vi "OSA20X_GetAttributes.vi"(0 "reference in":refnum<class "OSA.lvclass">, 1 "OnlyGetDvrReference(False)":bool, 5 "error in (no error)":errorcluster) -> (14 "reference out":refnum<class "OSA.lvclass">, 15 "Data":T1={"Stop"=FALSE, "dataType"=enum."interferogram", "spectrometerIdx"=0, "buffer size interferogram"=0, "interferogram"={"new"=FALSE, "plot_x_ min"=0.0, "plot_x_max"=0.0, "plot_y_min"=0.0, "plot_y_max"=0.0, "Graph Intrfrgrm"=refnum, "timeStamp"=0, "signal (%)"=0.0, "traces"=[], "traces idx last"=0}, "spectrum"={"new"=FALSE, "plot_x_min"=0.0, "plot_x_max"=0.0, "plot_unit_x"=enum."wavenr/cm", "plot_unit_y"=enum."ADC counts", "plot_y_min"=0.0, "plot_y_max"=0.0, "Graph Spectrum"=refnum, "timeStamp"=0, "X_VAL_OPTIONS"=enum."MIN_MAX", "traces"=[], "traces idx last"=0}, "Thorlabs_OSA_64.lvclass:queue_action.ctlqueue ref"=refnum, "action"=enum."none", "plot zoom step"=0.0, "buffer semaphore"=refnum, "acq stopped"=FALSE, "dataType active"=enum."interferogram", "temperature (degr C)"=0.0, "pressure (hPa)"=0.0, "rel humidity (%)"=0.0, "settings"={"resolution"=0, "sensitivity"=0, "Average"=FALSE, "average nr"=1, "apodisation"=enum."NONE", "acq delay (ms)"=500, "airMesure"=enum."TEMPERATURE", "wmtr on"=FALSE, "intfgrm_smooth_width"=0, "intfgrm_smooth_nrOfPasses"=0, "intfgrm_smooth"=enum."NONE", "phaseCorrection"=enum."NONE", "zeroFill"=0, "spectr_smooth"=enum."NONE", "spectr_smooth_width"=0, "spectr_smooth_nrOfPasses"=0, "resolution (/cm)"=0.0, "REF wavelength, (nm)"=0.0, "gain_idx"=0, "gainAuto"=FALSE, "gain_relative"=0.0, "PD sensitivity mode"=enum."cool: better sensitivity/noise floor", "PD senseMode implemented"=FALSE, "SensorTemperature implemented"=FALSE, "SensorPressure implemented"=FALSE, "SensorHumidity implemented"=FALSE, "attenuationAuto"=FALSE, "attenuationOnOff"=FALSE, "attenuationAvailable"=FALSE, "offsetAvailable"=FALSE, "offset"=0, "offset max"=0}, "peaks position"=[], "peaks width"=[], "peaks height"=[], "peaks max nr"=0, "peaks latest nr"=0, "peaks new"=FALSE, "power"=0.0, "power new"=FALSE, "path"="", "wavelength (WNr)"=0.0, "wavelength new"=FALSE, "buffer size spectrum"=0, "status"="", "vi reference"=refnum, "funcPointer"=0, "libraryPointer"=0, "singleAcquisition"=FALSE, "coherenceLength (cm)"=0.0, "coherenceLength new"=FALSE, "spectrometer model"="", "spectrometer serial nr"="", "peaks thld left"=[], "peaks thld right"=[], "coherenceLength error (cm)"=0.0, "ADC bits"=0, "peaks position centroid"=[], "peaks height centroid"=[], "OSA series"=enum."OSA200", "channel index spectrum"=0, "spectrometer rangeLow, (/cm)"=0.0, "spectrometer rangeHigh, (/cm)"=0.0, "channel index interferogram"=0} {"peaks height centroid" format="%.2f"; "peaks position centroid" format="%.2f"; "coherenceLength error (cm)" format="%.2f"; "peaks thld right" format="%.2f"; "peaks thld left" format="%.2f"; "coherenceLength (cm)" format="%.2f"; "wavelength (WNr)" format="%.2f"; "power" format="%.2f"; "peaks height" format="%.2f"; "peaks width" format="%.2f"; "peaks position" format="%.2f"; "settings"."REF wavelength, (nm)" format="%.2f"; "settings"."resolution (/cm)" format="%.2f"; "settings"."acq delay (ms)" step=200; "settings"."average nr" min=1 max=100 step=1; "rel humidity (%)" format="%.2f"; "pressure (hPa)" format="%.2f"; "temperature (degr C)" format="%.2f"; "plot zoom step" format="%.2f"; "spectrum"."plot_y_max" format="%.2f"; "spectrum"."plot_y_min" format="%.2f"; "spectrum"."plot_x_max" format="%.2f"; "spectrum"."plot_x_min" format="%.2f"; "interferogram"."plot_y_max" format="%.2f"; "interferogram"."plot_y_min" format="%.2f"; "interferogram"."plot_x_max" format="%.2f"; "interferogram"."plot_x_ min" format="%.2f"}, 17 "DataRef":refnum<data-value>, 19 "error out":errorcluster)   [LabVIEW 2010, in "OSA.lvclass"]
uses:
  OSA.lvclass
  protected/ObjectAttributes.ctl
  typeDef/acq_dataType.ctl
  private/graph_intensity.ctl
  typeDef/spectrum_x_unit.ctl
  typeDef/y_unit.ctl
  misc_examples/action_data.ctl
  typeDef/queue_action.ctl
  typeDef/apodisation.ctl
  typeDef/airMeasure.ctl
  _misc/Thorlabs_FTS_misc.llb/interferogram_smoothing.ctl
  typeDef/phaseCorrection.ctl
  _misc/Thorlabs_FTS_misc.llb/PDTemperatureMode.ctl
  typeDef/OSA_series.ctl
  OSA.lvclass/OSA.ctl
  OSA20X_misc.lvlib
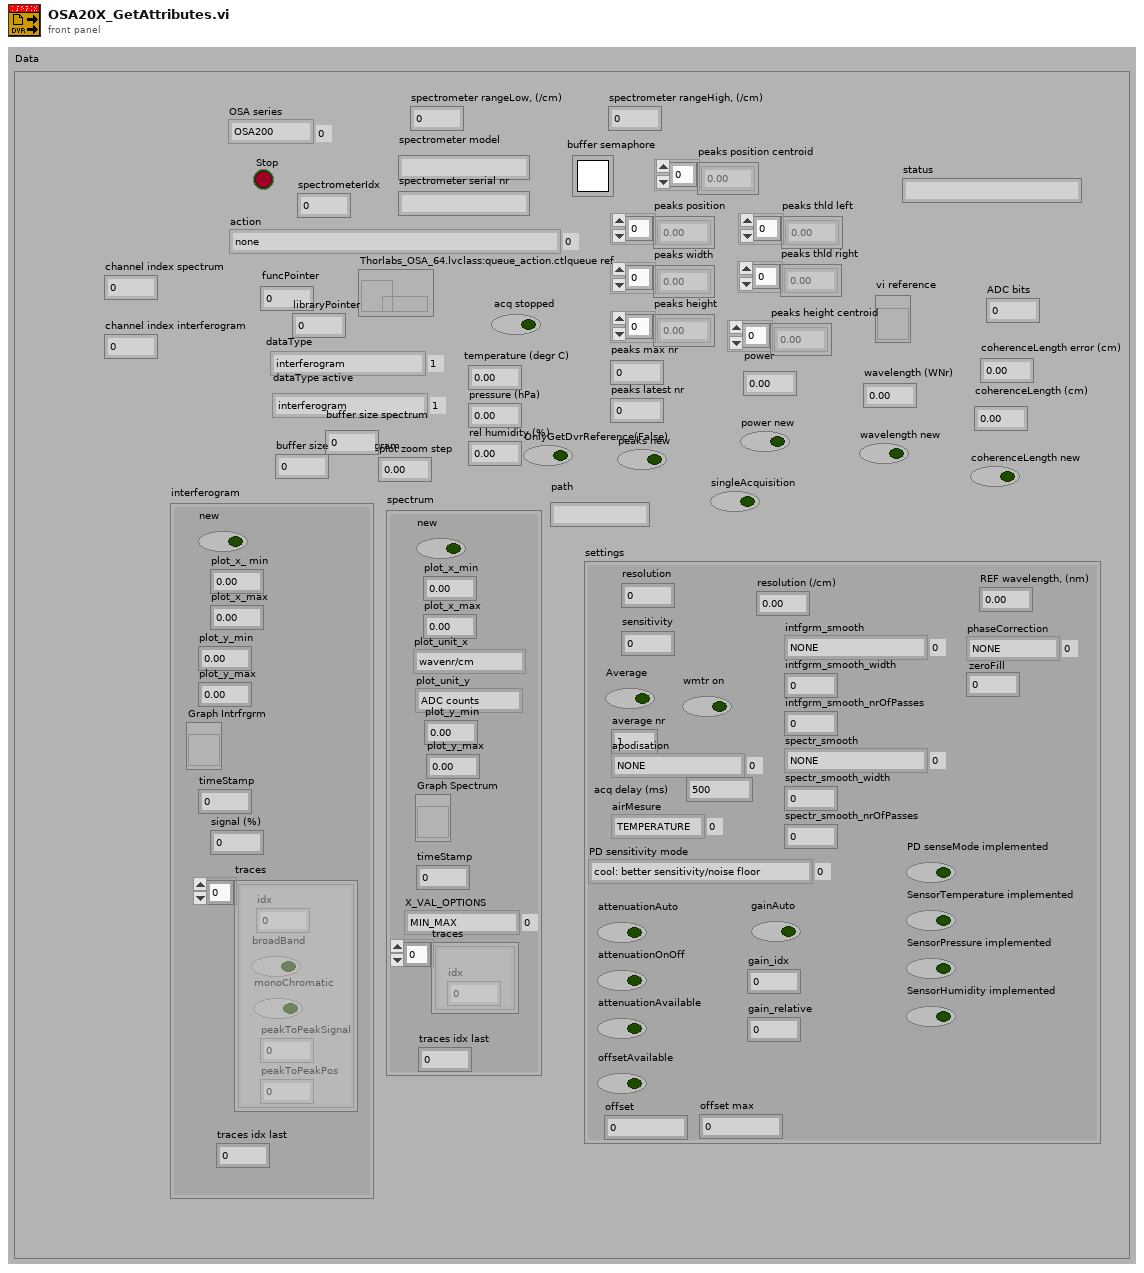
[diagram p1: front panel]
types:
  T1 = typedef "OSA.lvclass/ObjectAttributes.ctl" = cluster{"Stop":bool, "dataType":T2, "spectrometerIdx":u16, "buffer size interferogram":i32, "interferogram":cluster{"new":bool, "plot_x_ min":sgl, "plot_x_max":sgl, "plot_y_min":sgl, "plot_y_max":sgl, "Graph Intrfrgrm":T3, "timeStamp":u32, "signal (%)":dbl, "traces":cluster{"idx":u32, "broadBand":bool, "monoChromatic":bool, "peakToPeakSignal":dbl, "peakToPeakPos":dbl}[], "traces idx last":i32}, "spectrum":cluster{"new":bool, "plot_x_min":sgl, "plot_x_max":sgl, "plot_unit_x":T4, "plot_unit_y":T5, "plot_y_min":sgl, "plot_y_max":sgl, "Graph Spectrum":T3, "timeStamp":u32, "X_VAL_OPTIONS":enum16{"MIN_MAX", "ARRAY"}, "traces":cluster{"idx":u32}[], "traces idx last":i32}, "Thorlabs_OSA_64.lvclass:queue_action.ctlqueue ref":refnum<queue>, "action":T6, "plot zoom step":dbl, "buffer semaphore":T7, "acq stopped":bool, "dataType active":T2, "temperature (degr C)":sgl, "pressure (hPa)":sgl, "rel humidity (%)":sgl, "settings":cluster{"resolution":u16, "sensitivity":u16, "Average":bool, "average nr":u32, "apodisation":T8, "acq delay (ms)":u32, "airMesure":T9, "wmtr on":bool, "intfgrm_smooth_width":u16, "intfgrm_smooth_nrOfPasses":u16, "intfgrm_smooth":T10, "phaseCorrection":T11, "zeroFill":u8, "spectr_smooth":T10, "spectr_smooth_width":u16, "spectr_smooth_nrOfPasses":u16, "resolution (/cm)":sgl, "REF wavelength, (nm)":dbl, "gain_idx":u16, "gainAuto":bool, "gain_relative":dbl, "PD sensitivity mode":T12, "PD senseMode implemented":bool, "SensorTemperature implemented":bool, "SensorPressure implemented":bool, "SensorHumidity implemented":bool, "attenuationAuto":bool, "attenuationOnOff":bool, "attenuationAvailable":bool, "offsetAvailable":bool, "offset":i32, "offset max":u16}, "peaks position":sgl[], "peaks width":sgl[], "peaks height":sgl[], "peaks max nr":u32, "peaks latest nr":i32, "peaks new":bool, "power":dbl, "power new":bool, "path":string, "wavelength (WNr)":dbl, "wavelength new":bool, "buffer size spectrum":i32, "status":string, "vi reference":refnum<vi>, "funcPointer":u64, "libraryPointer":u64, "singleAcquisition":bool, "coherenceLength (cm)":dbl, "coherenceLength new":bool, "spectrometer model":string, "spectrometer serial nr":string, "peaks thld left":sgl[], "peaks thld right":sgl[], "coherenceLength error (cm)":dbl, "ADC bits":u16, "peaks position centroid":sgl[], "peaks height centroid":sgl[], "OSA series":T13, "channel index spectrum":u16, "spectrometer rangeLow, (/cm)":dbl, "spectrometer rangeHigh, (/cm)":dbl, "channel index interferogram":u16}
  T2 = typedef "OSA.lvclass/acq_dataType.ctl" = enum16{"none", "interferogram", "spectrum"}
  T3 = typedef "OSA.lvclass/graph_intensity.ctl" = refnum<vi>
  T4 = typedef "OSA.lvclass/spectrum_x_unit.ctl" = enum16{"wavenr/cm", "THz", "eV", "nm_air", "nm_vac"}
  T5 = typedef "OSA.lvclass/y_unit.ctl" = enum16{"ADC counts", "dBm pwr absolute", "dBm pwr density", "mW pwr absolute", "mW pwr density"}
  T6 = typedef "OSA.lvclass/queue_action.ctl" = enum16{"none", "stop", "GUI_plotInterferogram", "GUI_plotSpectrum", "GUI_plotInterferogramRescale", "GUI_plotSpectrumRescale", "GUI_plotInterferogramReset", "GUI_plotSpectrumReset", "GUI_plotInterferogramAutoScaleY", "GUI_plotSpectrumAutoScaleY", "GUI_plotInterferogramZoomOut", "GUI_plotSpectrumZoomOut", "GUI_plotInterferogramPane", "GUI_plotSpectrumPane", "GUI_plotInterferogramZoomMouse", "GUI_plotSpectrumZoomMouse", "GUI_spectrumChannelType", "GUI_channel", "ENVIRONMENT temperature", "ENVIRONMENT pressure", "MODE_resolution set", "MODE_resolution get", "MODE_sensitivity set", "MODE_sensitivity get", "MODE_PDTemperature set", "MODE_PDTemperature get", "REBOOT/RESET firmware", "ACQASYNC_acquireSingleSpectrum", "ACQASYNC_continuous start", "ACQASYNC_continuous stop\n", "ACQASYNC_get last interferogram", "ACQASYNC_get last spectrum", "ACQASYNC_get last waveNr", "ACQOPT_interferogram smoothing set", "ACQOPT_interferogram smoothing get", "ACQOPT_spectrum smoothing set", "ACQOPT_spectrum smoothing get", "ACQOPT_apodisation type set", "ACQOPT_apodisation type get", "ACQOPT_phase correction type set", "ACQOPT_phase correction type get", "ACQOPT_acqIntervall_set", "ACQOPT_acqIntervall_get", "ACQOPT_average spectrum set", "ACQOPT_average spectrum get", "ACQOPT_rolling average set", "ACQOPT_rolling average get", "ACQOPT_zero fill factor set", "ACQOPT_zero fill factor get", "ACQOPT_cycle counting set", "ACQOPT_cycle counting get", "ACQOPT_air measure option set", "ACQOPT_air measure option get", "ACQOPT_gainLevel auto get", "ACQOPT_gainLevel auto set", "ACQOPT_gainLevel get", "ACQOPT_gainLevel set", "ACQOPT_offset set", "ACQOPT_attenuator_auto_set", "ACQOPT_attenuator_set", "ACQOPT_getAll", "INSTRUMENT_PROPERTY_range_WaveNr_min", "INSTRUMENT_PROPERTY_range_WaveNr_max", "INSTRUMENT_PROPERTY_reference_wavelength_cm^-1", "INSTRUMENT_PROPERTY_samplesPerRefPeriod", "INSTRUMENT_PROPERTY_resolution_waveNrPercm", "INSTRUMENT_PROPERTY_availableGainLevels", "INSTRUMENT_PROPERTY_status", "CONVERT", "ANALYSE_POWER", "ANALYSE_PEAKS", "ANALYSE_WAVELENGTH", "ANALYSE_SPECTRUM", "ANALYSE_INTERFEROGRAM", "ANALYSE_COHERENCE_LENGTH", "MATH", "MATH_power", "MATH_peaks", "FILE", "miscellaneous"}
  T7 = typedef "Semaphore RefNum" = refnum<k1>
  T8 = typedef "OSA.lvclass/apodisation.ctl" = enum16{"NONE", "NORTON_BEER_WEAK", "NORTON_BEER_MEDIUM", "NORTON_BEER_STRONG", "TRIANGULAR", "COSINE", "HANN", "HAMMING", "BLACKMANHARRIS3", "BLACKMANHARRIS4", "GAUSSIAN"}
  T9 = typedef "OSA.lvclass/airMeasure.ctl" = enum16{"TEMPERATURE", "PRESSURE"}
  T10 = typedef "OSA20X_misc.lvlib/interferogram_smoothing.ctl" = enum16{"NONE", "BINOMIAL", "SAVITSKY_GOLAY", "FOURIER", "MOVING_AVERAGE", "GAUSSIAN"}
  T11 = typedef "OSA.lvclass/phaseCorrection.ctl" = enum16{"NONE", "MERTZ", "FORMAN", "MERTZ_FILE", "FORMAN_FILE", "FUTURE COMP."}
  T12 = typedef "OSA20X_misc.lvlib/PDTemperatureMode.ctl" = enum16{"cool: better sensitivity/noise floor", "warm: extended wl range"}
  T13 = typedef "OSA.lvclass/OSA_series.ctl" = enum16{"OSA200", "OSA300", "UNKNOWN"}
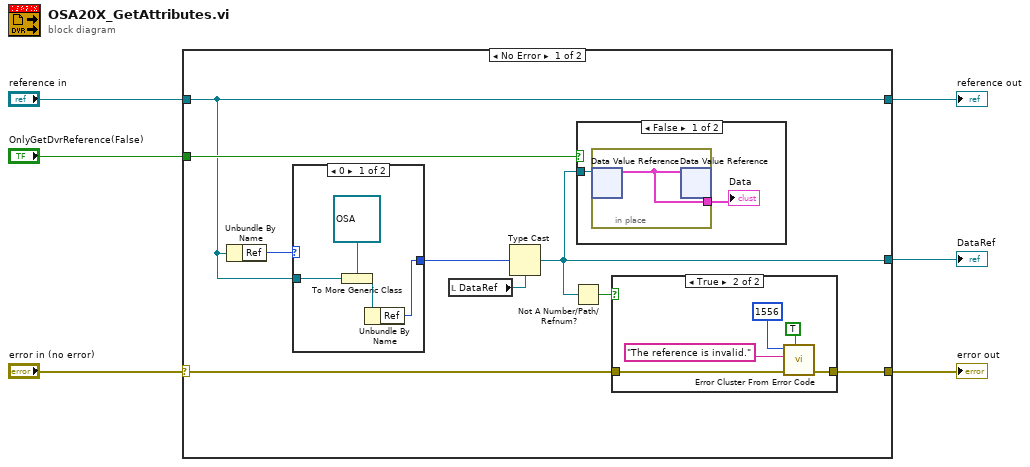
[diagram p0: block diagram]
diagram:
  n1 = case shown="No Error" "error in (no error)" {
    selector: "error in (no error)" -> [w12 w30]
    tunnel: [w10 w30] -> w5
    tunnel: [w8 w31] -> w3
    tunnel: "reference in" -> [w8 w31]
    tunnel: [w13 _] -> w2
    tunnel: "OnlyGetDvrReference(False)" -> [w14 _]
    frame No Error {
      n2 = Unbundle By Name(w8) -> ("Ref"=w9:u32)
      n3 = case shown="0" w9 {
        selector: w9 -> [_ w20]
        tunnel: w8 -> [w19 _]
        tunnel: [w16 w20] -> w7
        frame 0 {
          n4 = To More Generic Class(target class=refnum<class "OSA.lvclass"> refnum ("Thorlabs_OSA_64"), reference=w19) -> (generic class reference=w17:refnum<class "OSA.lvclass">)
          n5 = Unbundle By Name(w17) -> ("Ref"=w16:u32)
        }
        frame Default {
        }
      }
      n6 = local read "DataRef"() -> (w15:refnum<data-value>)
      n7 = Type Cast(type=w15, x=w7) -> (*(type *) &x=w13:refnum<data-value>)
      n8 = Not A Number/Path/Refnum?(number/path/refnum=w13) -> (NaN/Path/Refnum?=w11:bool)
      n9 = case shown="False" w14 {
        tunnel: w13 -> [w28 _]
        frame False {
          n10 = in-place {
            in-place-border: [w29] -> w27
            n11 = in-place-dvr #1(w28) -> (w29:T1)  [unwired: 1 out]
            n12 = in-place-dvr #1(w29) -> ()  [unwired: 2 out]
          }
          "Data" <- w27
        }
        frame True {
        }
      }
      n13 = case shown="True" w11 {
        tunnel: w12 -> [w21 w23]
        tunnel: [w21 w22] -> w10
        frame False {
        }
        frame True {
          n14 = call <vilib>:"Error Cluster From Error Code.vi"("show call chain? (False)"=TRUE, "error in (no error)"=w23, "error message (\"\")"="The reference is invalid." ("source"), "error code (0)"=1556 ("code")) -> ("error out"=w22:errorcluster)  [unwired: 5 in]
        }
      }
    }
    frame Error {
    }
  }
  "error out" <- w5
  "reference out" <- w3
  "DataRef" <- w2
